vi "Create_Time_Seq.vi"(9 "pulses":map{string, dbl}(c390), 10 "Channels and actions":map{string, i32}(c390), 11 "Array sequence in":cluster{"Timing 0":dbl[]}[](array[cluster])) -> (3 "Array out":cluster{"Timing 0":dbl[]}[][](array[cluster]))   [LabVIEW 2021]
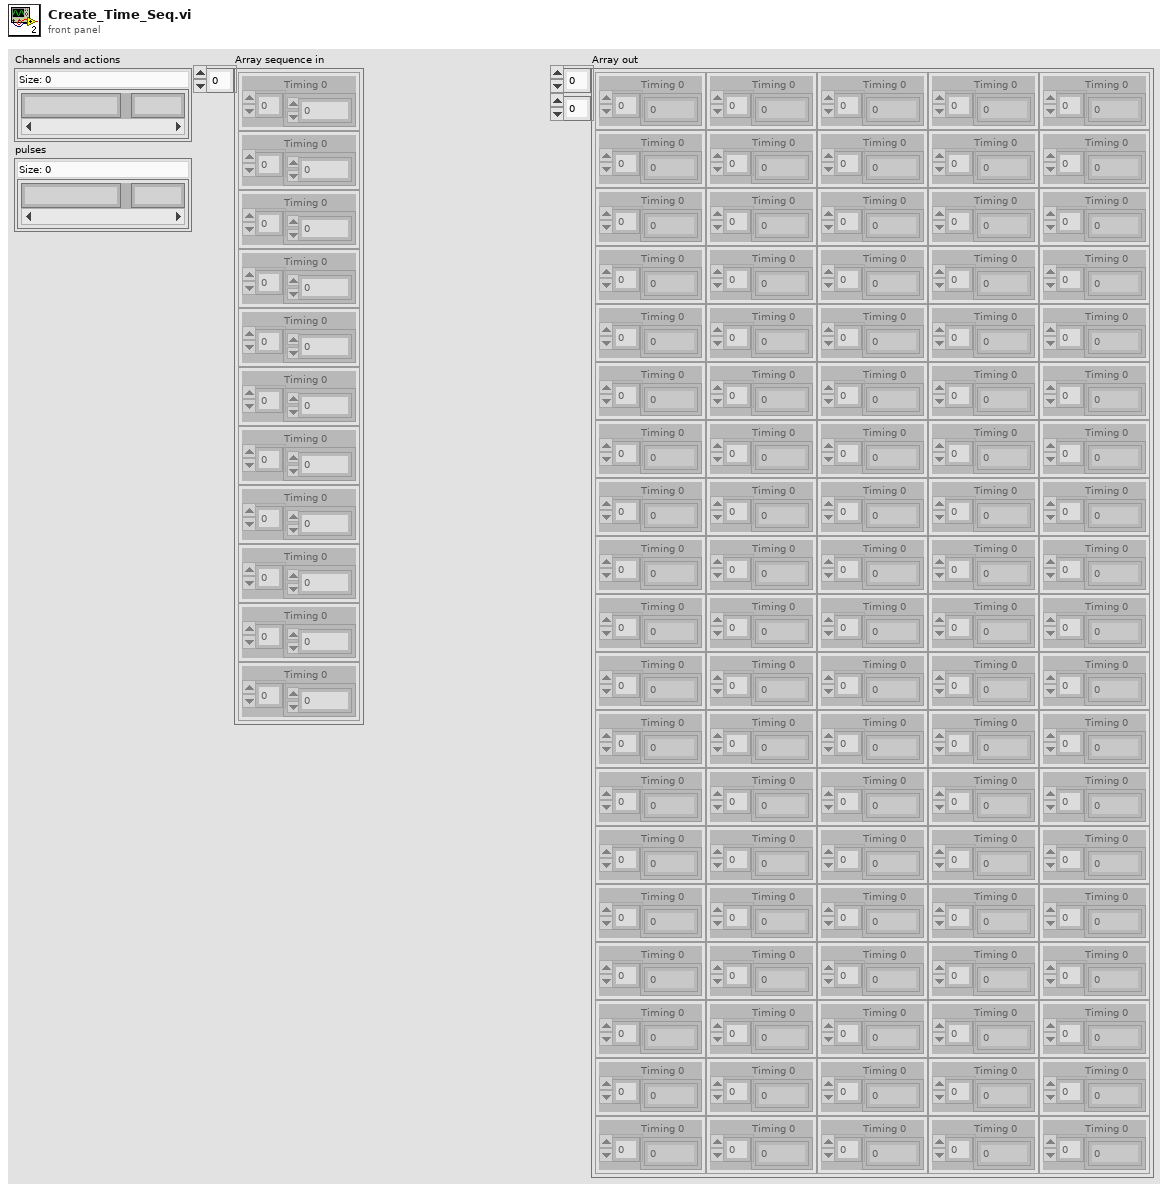
[diagram p1: front panel]
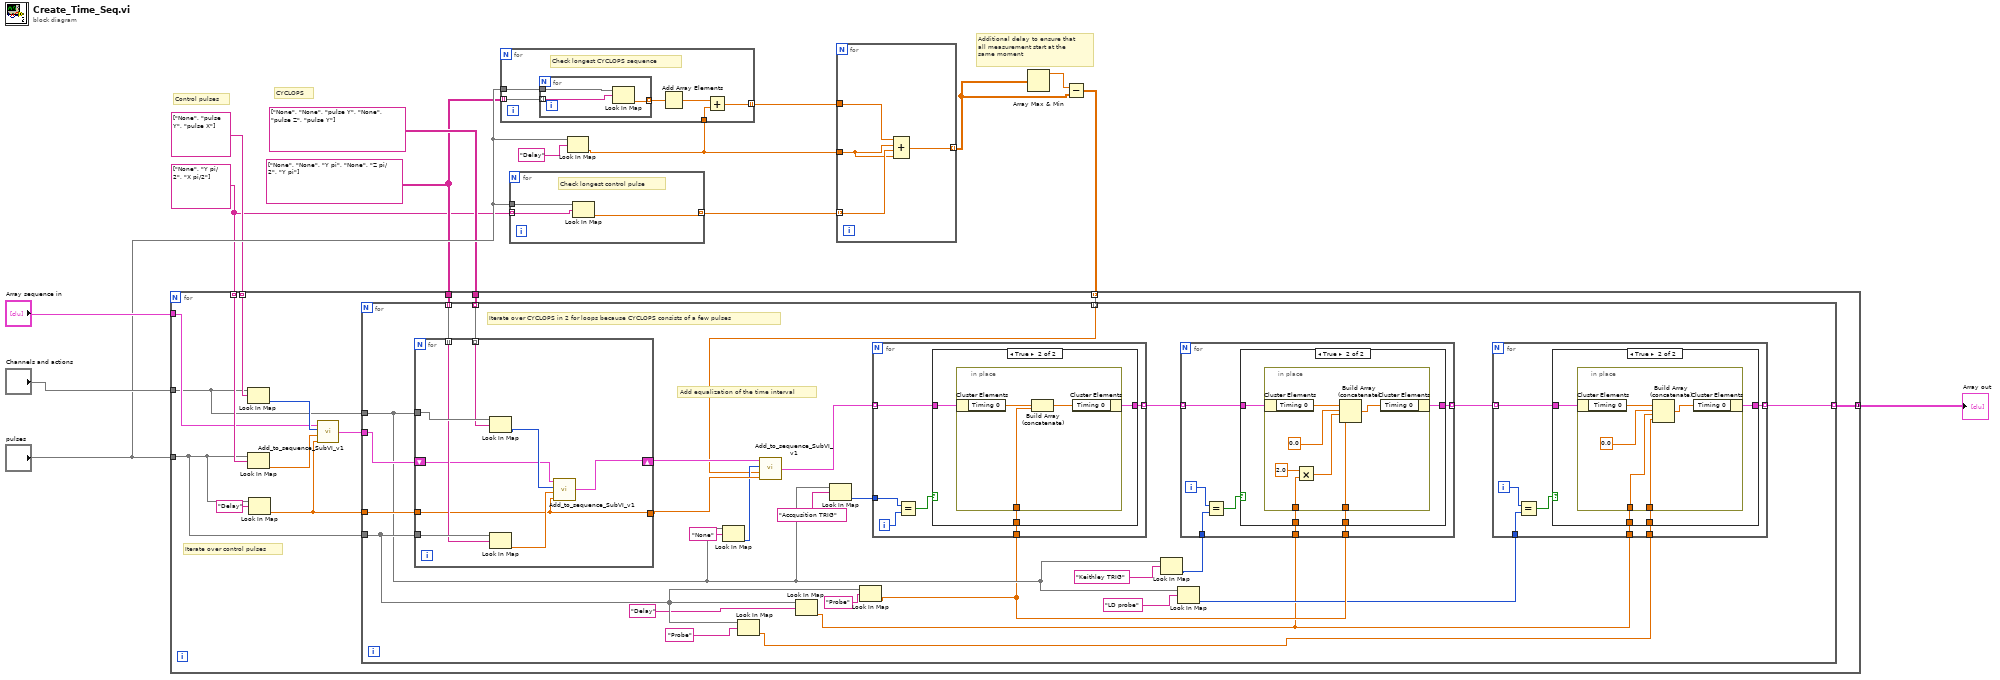
[diagram p0: block diagram]
diagram:
  w10 = string[][] [["None", "None"], ["Y pi", "None"], ["Z pi/2", "Y pi"]]
  w8 = string[] ["None", "Y pi/2", "X pi/2"]
  # "Additional delay to ensure that\nall measurement start at the\nsame moment"
  # "CYCLOPS"
  # "Control pulses"
  n1 = for {
    tunnel: "pulses" -> [w18]
    tunnel: w8 -> [w17] mode=indexing
    tunnel: [w16] -> w5 mode=indexing
    # "Check longest control pulse"
    n2 = Look In Map(map=w18, key=w17) -> (value=w16:dbl)  [unwired: 1 in, 1 out]
  }
  n3 = Look In Map(map="pulses", key="Delay") -> (value=w6:dbl)  [unwired: 1 in, 1 out]
  n4 = for {
    tunnel: "pulses" -> [w24]
    tunnel: w10 -> [w23] mode=indexing
    tunnel: w6 -> [w20]
    tunnel: [w19] -> w7 mode=indexing
    # "Check longest CYCLOPS sequence"
    n5 = for {
      tunnel: w24 -> [w27]
      tunnel: w23 -> [w26] mode=indexing
      tunnel: [w25] -> w22 mode=indexing
      n6 = Look In Map(map=w27, key=w26) -> (value=w25:dbl)  [unwired: 1 in, 1 out]
    }
    n7 = Add Array Elements(numeric array=w22) -> (sum=w21:dbl)
    n8 = Add(x=w21, y=w20) -> (x+y=w19:dbl)
  }
  n9 = for {
    tunnel: w7 -> [w31]
    tunnel: w6 -> [w29]
    tunnel: w5 -> [w30] mode=indexing
    tunnel: [w28] -> w2 mode=indexing
    n10 = Compound Arithmetic op=unknown(w31, w29, w30, w29) -> (w28:dbl[])
  }
  n11 = Array Max & Min(array=w2) -> (max value=w4:dbl)  [unwired: 3 out]
  n12 = Subtract(x=w4, y=w2) -> (x-y=w3:dbl[][])
  n13 = for {
    tunnel: "Channels and actions" -> [w39]
    tunnel: "pulses" -> [w37]
    tunnel: w8 -> [w45] mode=indexing
    tunnel: string[] ["None", "pulse Y", "pulse X"] -> [w44] mode=indexing
    tunnel: "Array sequence in" -> [w40]
    tunnel: w10 -> [w36]
    tunnel: string[][] [["None", "None"], ["pulse Y", "None"], ["pulse Z", "pulse Y"]] -> [w34]
    tunnel: w3 -> [w33] mode=indexing
    tunnel: [w32] -> w1 mode=concatenating
    # "Iterate over control pulses"
    n14 = Look In Map(map=w39, key=w44) -> (value=w41:i32)  [unwired: 1 in, 1 out]
    n15 = Look In Map(map=w37, key=w45) -> (value=w42:dbl)  [unwired: 1 in, 1 out]
    n16 = Look In Map(map=w37, key="Delay") -> (value=w35:dbl)  [unwired: 1 in, 1 out]
    n17 = call "Add_to_sequence_SubVI_v1.vi"("Delay [us]"=w35, "Pulse length [us]"=w42, "Channel number"=w41, "Array sequence in"=w40) -> ("Array sequence out"=w38:cluster{"Timing 0":dbl[]}[])
    n18 = for {
      tunnel: w39 -> [w54]
      tunnel: w38 -> [w72]
      tunnel: w37 -> [w61]
      tunnel: w36 -> [w71] mode=indexing
      tunnel: w35 -> [w70]
      tunnel: w34 -> [w69] mode=indexing
      tunnel: w33 -> [w47] mode=indexing
      tunnel: [w46] -> w32 mode=indexing
      # "Add equalization of the time interval"
      # "Iterate over CYCLOPS in 2 for loops because CYCLOPS consists of a few pulses"
      n19 = for {
        tunnel: w54 -> [w130]
        shift-right: [w122] -> w68
        shift-left: w72 -> [w123]
        tunnel: w61 -> [w129]
        tunnel: w71 -> [w128] mode=indexing
        tunnel: [w126] -> w67
        tunnel: w70 -> [w126]
        tunnel: w69 -> [w125] mode=indexing
        n20 = Look In Map(map=w130, key=w125) -> (value=w124:i32)  [unwired: 1 in, 1 out]
        n21 = Look In Map(map=w129, key=w128) -> (value=w127:dbl)  [unwired: 1 in, 1 out]
        n22 = call "Add_to_sequence_SubVI_v1.vi"("Delay [us]"=w126, "Pulse length [us]"=w127, "Channel number"=w124, "Array sequence in"=w123) -> ("Array sequence out"=w122:cluster{"Timing 0":dbl[]}[])
      }
      n23 = Look In Map(map=w54, key="None") -> (value=w65:i32)  [unwired: 1 in, 1 out]
      n24 = Look In Map(map=w61, key="Probe") -> (value=w48:dbl)  [unwired: 1 in, 1 out]
      n25 = call "Add_to_sequence_SubVI_v1.vi"("Delay [us]"=w67, "Pulse length [us]"=w47, "Channel number"=w65, "Array sequence in"=w68) -> ("Array sequence out"=w62:cluster{"Timing 0":dbl[]}[])
      n26 = Look In Map(map=w61, key="Delay") -> (value=w49:dbl)  [unwired: 1 in, 1 out]
      n27 = Look In Map(map=w54, key="Accqusition TRIG") -> (value=w63:i32)  [unwired: 1 in, 1 out]
      n28 = Look In Map(map=w61, key="Probe") -> (value=w52:dbl)  [unwired: 1 in, 1 out]
      n29 = for {
        tunnel: w63 -> [w113]
        tunnel: w62 -> [w111] mode=indexing
        tunnel: w52 -> [w110]
        tunnel: [w109] -> w57 mode=indexing
        i -> [w112]
        n30 = Equal?(x=w113, y=w112) -> (x = y?=w114:bool)
        n31 = case shown="True" w114 {
          tunnel: w111 -> [w115 w117]
          tunnel: w110 -> [_ w118]
          tunnel: [w115 w116] -> w109
          frame False {
          }
          frame True {
            n32 = in-place {
              in-place-border: w118 -> [w121]
              n33 = in-place-cluster #1(w117) -> ("Timing 0"=w120:dbl[])
              n34 = Build Array (concatenate)(w120, w121) -> (w119:dbl[])
              n35 = in-place-cluster #1("Timing 0"=w119) -> (w116:cluster{"Timing 0":dbl[]})
            }
          }
        }
      }
      n36 = Look In Map(map=w54, key="Keithley TRIG") -> (value=w55:i32)  [unwired: 1 in, 1 out]
      n37 = Look In Map(map=w54, key="LD probe") -> (value=w50:i32)  [unwired: 1 in, 1 out]
      n38 = for {
        tunnel: w57 -> [w95] mode=indexing
        tunnel: [w94] -> w51 mode=indexing
        tunnel: w55 -> [w92]
        tunnel: w52 -> [w91]
        tunnel: w49 -> [w90]
        i -> [w93]
        n39 = Equal?(x=w93, y=w92) -> (x = y?=w96:bool)
        n40 = case shown="True" w96 {
          tunnel: w95 -> [w97 w101]
          tunnel: [w97 w100] -> w94
          tunnel: w91 -> [_ w99]
          tunnel: w90 -> [_ w98]
          frame False {
          }
          frame True {
            n41 = in-place {
              in-place-border: w99 -> [w107]
              in-place-border: w98 -> [w106]
              n42 = in-place-cluster #2(w101) -> ("Timing 0"=w108:dbl[])
              n43 = Multiply(x=2.0, y=w106) -> (x*y=w104:dbl)
              n44 = Build Array (concatenate)(w108, 0.0 ("x"), w104, w107) -> (w102:dbl[])
              n45 = in-place-cluster #2("Timing 0"=w102) -> (w100:cluster{"Timing 0":dbl[]})
            }
          }
        }
      }
      n46 = for {
        tunnel: w51 -> [w78] mode=indexing
        tunnel: [w77] -> w46 mode=indexing
        tunnel: w50 -> [w75]
        tunnel: w49 -> [w74]
        tunnel: w48 -> [w73]
        i -> [w76]
        n47 = Equal?(x=w76, y=w75) -> (x = y?=w79:bool)
        n48 = case shown="True" w79 {
          tunnel: w78 -> [w80 w84]
          tunnel: [w80 w83] -> w77
          tunnel: w74 -> [_ w82]
          tunnel: w73 -> [_ w81]
          frame False {
          }
          frame True {
            n49 = in-place {
              in-place-border: w82 -> [w86]
              in-place-border: w81 -> [w85]
              n50 = in-place-cluster #3(w84) -> ("Timing 0"=w89:dbl[])
              n51 = Build Array (concatenate)(w89, 0.0 ("x"), w86, w85) -> (w87:dbl[])
              n52 = in-place-cluster #3("Timing 0"=w87) -> (w83:cluster{"Timing 0":dbl[]})
            }
          }
        }
      }
    }
  }
  "Array out" <- w1
